vi "Write Is Connected.vi"(8 "error in (no error)":errorcluster, 10 "Is Connected":bool, 11 "MotorDrive in":refnum<class "MotorDrive.lvclass">) -> (0 "error out":errorcluster, 3 "MotorDrive out":refnum<class "MotorDrive.lvclass">)   [LabVIEW 2016, in "MotorDrive.lvclass"]
uses:
  MotorDrive.lvclass
  MotorDrive.lvclass/MotorDrive.ctl
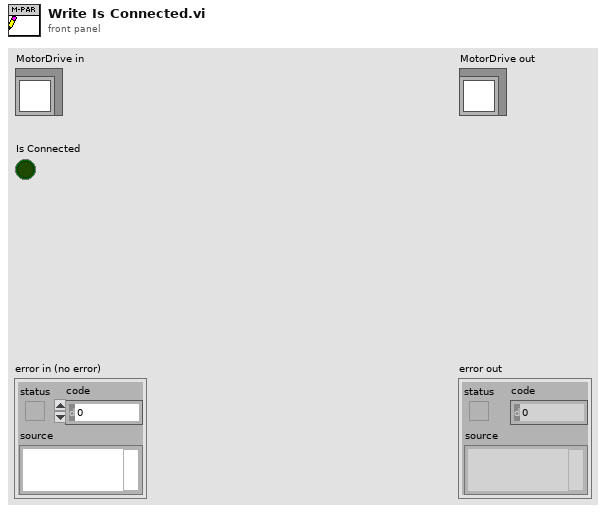
[diagram p1: front panel]
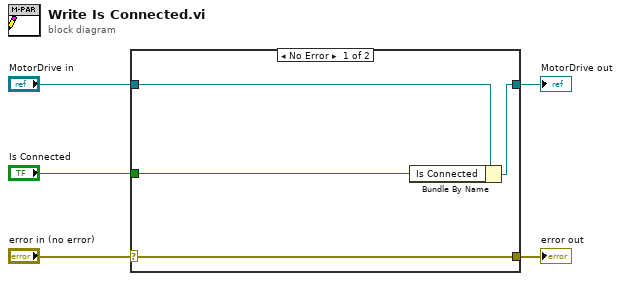
[diagram p0: block diagram]
diagram:
  n1 = case shown="No Error" "error in (no error)" {
    selector: "error in (no error)" -> [w9 w10]
    tunnel: [w9 w10] -> w4
    tunnel: [w7 w11] -> w2
    tunnel: "MotorDrive in" -> [w8 w11]
    tunnel: "Is Connected" -> [w6 _]
    frame No Error {
      n2 = Bundle By Name(cluster=w8, "Is Connected"=w6) -> (w7:refnum<class "MotorDrive.lvclass">)
    }
    frame Error {
    }
  }
  "error out" <- w4
  "MotorDrive out" <- w2
